vi "Pad1d array with wrap around data (dbl).vi"(9 "Pad Size in":i32, 11 "Data In":dbl[](array[numeric])) -> (1 "Pad Size":i32, 2 "Original Size":i32, 3 "Padded Array":dbl[](array[numeric]))   [LabVIEW 2013]
doc: "Wraps data by specified percent"
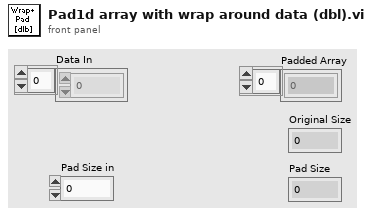
[diagram p1: front panel]
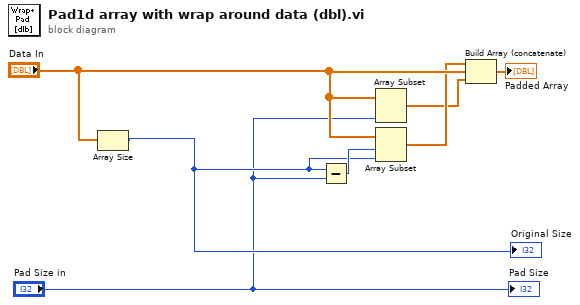
[diagram p0: block diagram]
diagram:
  n1 = Array Size(array="Data In") -> (size(s)=w2:i32)
  "Original Size" <- w2
  n2 = Subtract(x=w2, y="Pad Size in") -> (x-y=w3:i32)
  n3 = Array Subset(array="Data In", length="Pad Size in") -> (w4:dbl[])  [unwired: 1 in]
  n4 = Array Subset(array="Data In", index=w3, length=w2) -> (w5:dbl[])
  n5 = Build Array (concatenate)(w5, "Data In", w4) -> (→"Padded Array":dbl[])
  "Pad Size" <- "Pad Size in"
